vi "Update Visibility.vi"(8 "error in (no error)":errorcluster, 10 "Visible":bool, 11 "GUI Helper in":refnum<class "GUI Helper.lvclass">) -> (0 "error out":errorcluster, 3 "GUI Helper out":refnum<class "GUI Helper.lvclass">)   [LabVIEW 2020, in "VolatusGUI.lvlib" / "GUI Helper.lvclass"]
uses:
  GUI Helper.lvclass
  Visibility Data.ctl
  GUI Helper.lvclass/GUI Helper.ctl
  Volatus/MessageQ/MessageQ.lvclass/MessageQ.ctl
  VolatusGUI.lvlib
  Volatus/MessageQ/MessageQ.lvclass
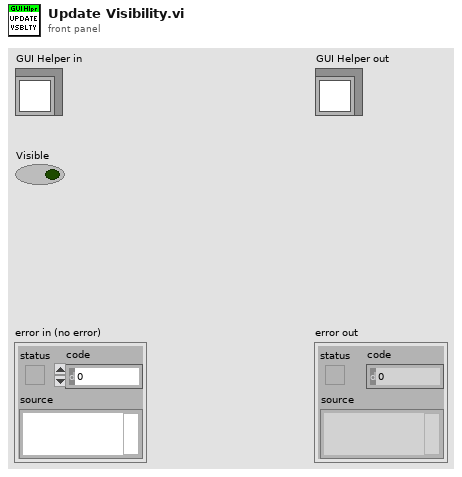
[diagram p1: front panel]
types:
  T1 = typedef "VolatusGUI.lvlib/Visibility Data.ctl" = cluster{"GUI ID":string, "Visible":bool}
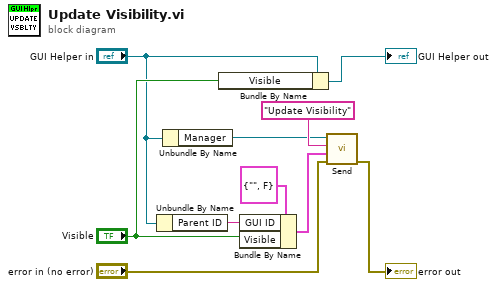
[diagram p0: block diagram]
diagram:
  n1 = Unbundle By Name("GUI Helper in") -> ("Parent ID"=w1:string)
  n2 = Unbundle By Name("GUI Helper in") -> ("Manager"=w7:refnum<class "MessageQ.lvclass">)
  n3 = Bundle By Name(cluster="GUI Helper in", "Visible"="Visible") -> (→"GUI Helper out":refnum<class "GUI Helper.lvclass">)
  n4 = Bundle By Name(cluster=T1 {"GUI ID"="", "Visible"=FALSE} ("Visibility Data"), "GUI ID"=w1, "Visible"="Visible") -> (w9:T1)
  n5 = call "Send.vi"("error in (no error)"="error in (no error)", "Data"=w9, "ID"="Update Visibility", "MessageQ in"=w7) -> ("error out"=→"error out":errorcluster)  [unwired: 6 in, 1 out]
